vi "Main.vi"() -> ()   [LabVIEW 2019]
panel:
  in  "Tab Control":enum32{"Page 1", "Page 2"}(tab)
  out "Waveform Chart 2":cluster{dbl, dbl, dbl}(graph)
  in  "VISA resource name":refnum<visa-resource-name>="COM3"
  in  "termination char\n(0xA = '\\n' = LF)":u8=13 format="%.0x"
  in  "Recieve Data":bool
  out "Thermometer":dbl(slide) scale=0.0..100.0
  out "Waveform Chart":T1(graph)
  in  "physical channels":tag="PXI1Slot2/ai2"
  in  "resistance configuration":i32(ring)=2 items=["2-Wire"=2, "3-Wire"=3, "4-Wire"=4]
  in  "valor":i32
  in  "stop":bool
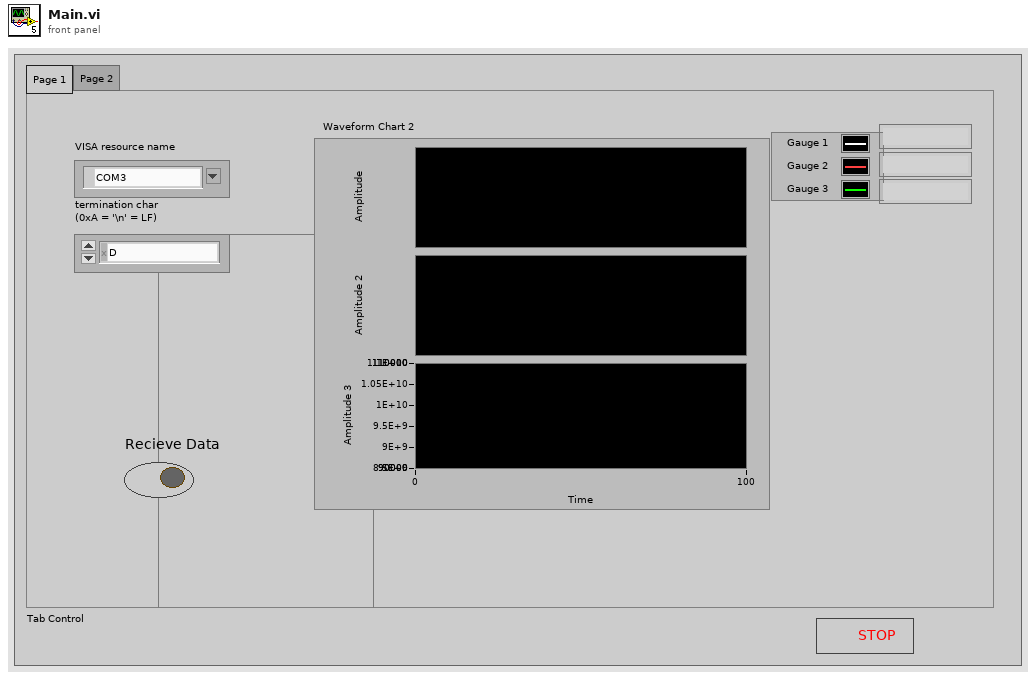
[diagram p1: front panel]
types:
  T1 = cluster{"data[0]":dbl, "data[1]":dbl, "data[2]":dbl, "data[3]":dbl, "data[4]":dbl, "data[5]":dbl, "data[6]":dbl, "data[7]":dbl, "data[8]":dbl, "data[9]":dbl, "data[10]":dbl, "data[11]":dbl, "data[12]":dbl, "data[13]":dbl, "data[14]":dbl, "data[15]":dbl, "data[16]":dbl, "data[17]":dbl, "data[18]":dbl, "data[19]":dbl}
  T2 = enum16{"open", "replace", "create", "open or create", "replace or create", "replace or create with confirmation"}
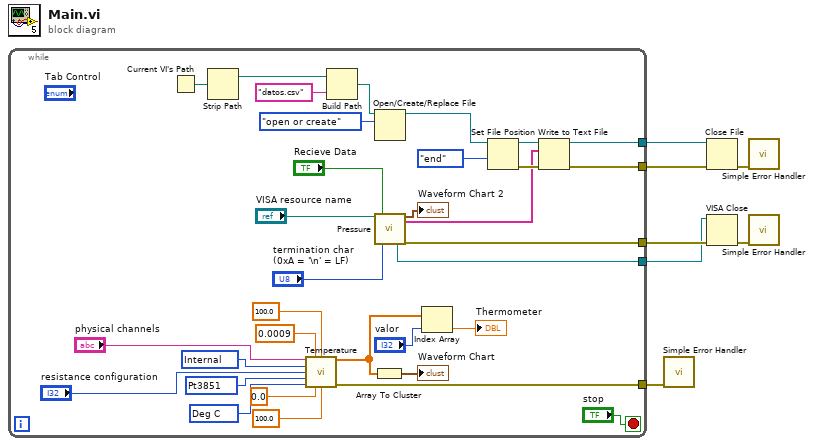
[diagram p0: block diagram]
diagram:
  n1 = while {
    tunnel: [w35] -> w7
    tunnel: [w34] -> w6
    tunnel: [w33] -> w4
    tunnel: [w22] -> w2
    tunnel: [w21] -> w1
    stop <- "stop" stop-if-true
    w12 = 10143 items=["Deg C"=10143, "Deg F"=10144, "Kelvins"=10325, "Deg R"=10145, "From Custom Scale"=10065] ("units")
    w13 = 10071 items=["Pt3750"=12481, "Pt3851"=10071, "Pt3911"=12482, "Pt3916"=10069, "Pt3920"=10053, "Pt3928"=12483, "Custom"=10137] ("rtd type")
    w14 = 10200 items=["Internal"=10200, "External"=10167, "None"=10230] ("current excitation source")
    n2 = Current VI's Path() -> (path=w29:path)
    n3 = Strip Path(path=w29) -> (stripped path=w30:path)  [unwired: 1 out]
    n4 = call "Temperature.vi"("physical channels"="physical channels", "current excitation value"=0.0009, "r0"=100.0, "current excitation source"=w14, "resistance configuration"="resistance configuration", "rtd type"=w13, "units"=w12, "minimum value"=0.0, "maximum value"=100.0) -> ("data"=w17:dbl[], "error out"=w33:errorcluster)  [unwired: 5 in]
    n5 = Build Path(base path=w30, name or relative path="datos.csv") -> (appended path=w31:path)
    n6 = Array To Cluster(array=w17) -> (cluster=→"Waveform Chart":T1)
    n7 = Open/Create/Replace File(file path (use dialog)=w31, operation (0:open)=T2."open or create") -> (refnum out=w32:refnum<file>)  [unwired: 4 in, 2 out]
    n8 = call "Pressure.vi"("VISA resource name"="VISA resource name", "Recieve Data"="Recieve Data", "termination char\n(0xA = '\\n' = LF)"="termination char\n(0xA = '\\n' = LF)") -> ("VISA resource name out"=w34:refnum<visa-resource-name>, "output cluster"=→"Waveform Chart 2":cluster{dbl, dbl, dbl}, "output array"=w23:string[], "error out"=w35:errorcluster)  [unwired: 10 in, 3 out]
    n9 = Index Array(array=w17, index="valor") -> (element=→"Thermometer":dbl)
    n10 = Set File Position(refnum=w32, from (0:start)=enum16{"start", "end", "current"}."end") -> (refnum out=w25:refnum<file>, error out=w24:errorcluster)  [unwired: 2 in]
    n11 = Write to Text File(file (use dialog)=w25, text=w23, error in=w24) -> (refnum out=w22:refnum<file>, error out=w21:errorcluster)  [unwired: 1 in, 1 out]
  }
  n12 = call <vilib>:"Simple Error Handler.vi"("error in (no error)"=w4) -> ()  [unwired: 4 in, 5 out]
  n13 = Close File(refnum=w2, error in=w1) -> (error out=w3:errorcluster)  [unwired: 1 out]
  n14 = VISA Close(VISA resource name=w6, error in (no error)=w7) -> (error out=w5:errorcluster)
  n15 = call <vilib>:"Simple Error Handler.vi"("error in (no error)"=w3) -> ()  [unwired: 1 in, 8 out]
  n16 = call <vilib>:"Simple Error Handler.vi"("error in (no error)"=w5) -> ()  [unwired: 4 in, 5 out]
